vi "Main.vi"(11 "Module Admin":refnum<class "Delacor_lib_QMH_Module Admin.lvclass">) -> ()   [LabVIEW 2025, in "Data Logger v2.lvlib"]
doc: "This template is based from the Queued Message Handler design pattern and the Queued Message Handler Project Template that ships with LabVIEW 2014.\n\nThe main difference is that the Queue is private to this module and communication between modules is done via Broadcast and Request events.\n\nRequest events are wrapped via public API methods and are handled in the Event handler loop in this VI.\nAny module can register for Broadcast events sent by this module.\n\nThe Event Handling Loop generates messages based on user interface actions.\n\nThe Message Handling Loop processes messages generated by the Event Handling Loop, or by other messages. The messages are string values, so new messages can be added easily to the Message Cases case structure in the Message Handling Loop. Each message cluster can also provide an optional value for Message Data, which is a variant that can be converted to whatever message-specific data is required.\n_____\nBased on Delacor QMH Project Template 3.1.0.34.\n\n<b>Note:</b> This VI was modified by the <b>Validate DQMH Module</b> tool to call the Release Message Queue VI in the top-level Error case.\n\n<b>Note:</b> This VI was modified by the <b>Validate DQMH Module</b> tool to add a call to the Error Reported VI at the end of the 'Exit' MHL frame.\n\n<b>Note:</b> This VI was modified by the <b>Validate DQMH Module</b> tool to wrap the FP.Open method in the module close code with a Conditional Disable Structure so it does not execute when the Main VI is running as a built EXE."
uses:
  Data Logger v2.lvlib
  <vilib>/Delacor/Delacor QMH/Libraries/Module Admin_class/Delacor_lib_QMH_Module Admin.lvclass
  <vilib>/MGI/Panel Manager/Panel/Panel/Panel.lvclass
  <vilib>/Utility/miscctls.llb/LVPointTypeDef.ctl
  Module Data--cluster.ctl
  <vilib>/Delacor/Delacor QMH/Libraries/Message Queue_class/Delacor_lib_QMH_Message Queue.lvclass/Delacor_lib_QMH_Message Queue.ctl
  Stop Argument--cluster.ctl
  <vilib>/Delacor/Delacor QMH/Libraries/Module Admin_class/Delacor_lib_QMH_Module Admin.lvclass/Delacor_lib_QMH_Module Admin.ctl
  Create New TDMS Log File Argument--cluster.ctl
  Write 2D Array to TDMS Log File Argument--cluster.ctl
  Write TDMS 2D Array Parameters--cluster.ctl
  Close TDMS File Argument--cluster.ctl
  Write TDMS 2D String Array Argument--cluster.ctl
  Write TDMS 2D String Array Parameters--cluster.ctl
  Set Root Folder Path Argument--cluster.ctl
  Create New TDMS Log File (Relative Path) Argument--cluster.ctl
  Set Properties Argument--cluster.ctl
  <vilib>/Delacor/Delacor QMH/Libraries/Message Queue_class/Delacor_lib_QMH_Enqueue Message (Single).vi
  <vilib>/Delacor/Delacor QMH/Libraries/Module Admin_class/Delacor_lib_QMH_Get External Launch.vi
  <vilib>/Utility/error.llb/Error Cluster From Error Code.vi
  <vilib>/ErrorRing/Error Ring.xnode
  <vilib>/Delacor/Delacor QMH/Libraries/Message Queue_class/Delacor_lib_QMH_Message Queue.lvclass
  <vilib>/MGI/Panel Manager/Panel/Panel Helper/Panel Helper.lvclass
panel:
  in  "Panel":refnum<class "Panel.lvclass">
  in  "Simulate MHL Error":bool
  in  "Simulate EHL Error":bool
  out "error out":errorcluster
  out "Status":string
  # "Other QMH Modules communicate with this Module via its Public API (wrappers for its Request Events).\n\nThis Module communicates with other Modules via its Broadcast Events.\nAny module that wants to get these messages, just registers for this module's Broadcast events."
  # "This is a template that creates a DQMH Singleton using the MGI Panel Manager Framwork.\n\nImplement your user interface on this front panel. The Panel Manager Framework will manage showing and hiding the panel in the appropriate spot. \n\nSee the block diagram for more information on how to use this template."
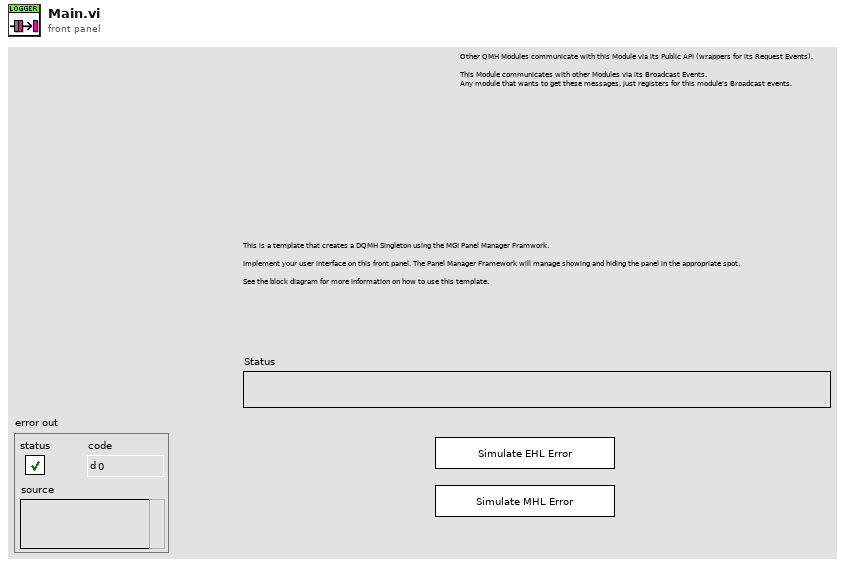
[diagram p1: front panel]
types:
  T1 = typedef "LVPointTypeDef.ctl" = cluster{"Horizontal":i16, "Vertical":i16}
  T2 = typedef "Data Logger v2.lvlib/Request Events--cluster.ctl" = cluster{"Stop Module":refnum<user-event>, "Show Panel":refnum<user-event>, "Hide Panel":refnum<user-event>, "Get Module Execution Status":refnum<user-event>, "Show Diagram":refnum<user-event>, "Change Panel":refnum<user-event>, "Create New TDMS Log File":refnum<user-event>, "Write 2D Array to TDMS Log File":refnum<user-event>, "Close TDMS File":refnum<user-event>, "Write TDMS 2D String Array":refnum<user-event>, "Set Root Folder Path":refnum<user-event>, "Create New TDMS Log File (Relative Path)":refnum<user-event>, "Set Properties":refnum<user-event>}
  T3 = typedef "Panel.lvlib/Panel Helper.lvclass/Panel Events.ctl" = cluster{"My Panel":refnum<user-event>, "Top Level Initialized":refnum<user-event>}
  T4 = typedef "Data Logger v2.lvlib/Module Data--cluster.ctl" = cluster{"Status":string, "tdms file":refnum<k34>, "State":enum16{"Idle", "Logging"}, "Root Folder Path":path}
  T5 = typedef "Data Logger v2.lvlib/Stop Argument--cluster.ctl" = cluster{"Origin":string, "Exit via Stop Module Req?":bool, "Wait for Module to stop?":bool}
  T6 = typedef "Data Logger v2.lvlib/Create New TDMS Log File Argument--cluster.ctl" = cluster{"File Path (inc. Filename)":path}
  T7 = typedef "Data Logger v2.lvlib/Write 2D Array to TDMS Log File Argument--cluster.ctl" = cluster{"TDMS Write 2D Array Parameters":T8}
  T8 = typedef "Data Logger v2.lvlib/Write TDMS 2D Array Parameters--cluster.ctl" = cluster{"Group":string, "Channel Names":string[], "Data":dbl[][]}
  T9 = typedef "Data Logger v2.lvlib/Close TDMS File Argument--cluster.ctl" = cluster{"Boolean":bool}
  T10 = typedef "Data Logger v2.lvlib/Write TDMS 2D String Array Argument--cluster.ctl" = cluster{"TDMS Write 2D String Array Parameters":T11}
  T11 = typedef "Data Logger v2.lvlib/Write TDMS 2D String Array Parameters--cluster.ctl" = cluster{"Group":string, "Channel Names":string[], "Data":string[][]}
  T12 = typedef "Data Logger v2.lvlib/Set Root Folder Path Argument--cluster.ctl" = cluster{"Root Folder Path":path}
  T13 = typedef "Data Logger v2.lvlib/Create New TDMS Log File (Relative Path) Argument--cluster.ctl" = cluster{"Filename":string}
  T14 = typedef "Data Logger v2.lvlib/Set Properties Argument--cluster.ctl" = cluster{"Property names":string[], "Property values":variant[], "Group name":string, "Channel name":string}
  T15 = enum32{"invalid lock state", "Not Locked", "Locked (No Password)", "Password-protected"}
  T16 = enum16{"open", "open or create", "create or replace", "create", "open (read-only)"}
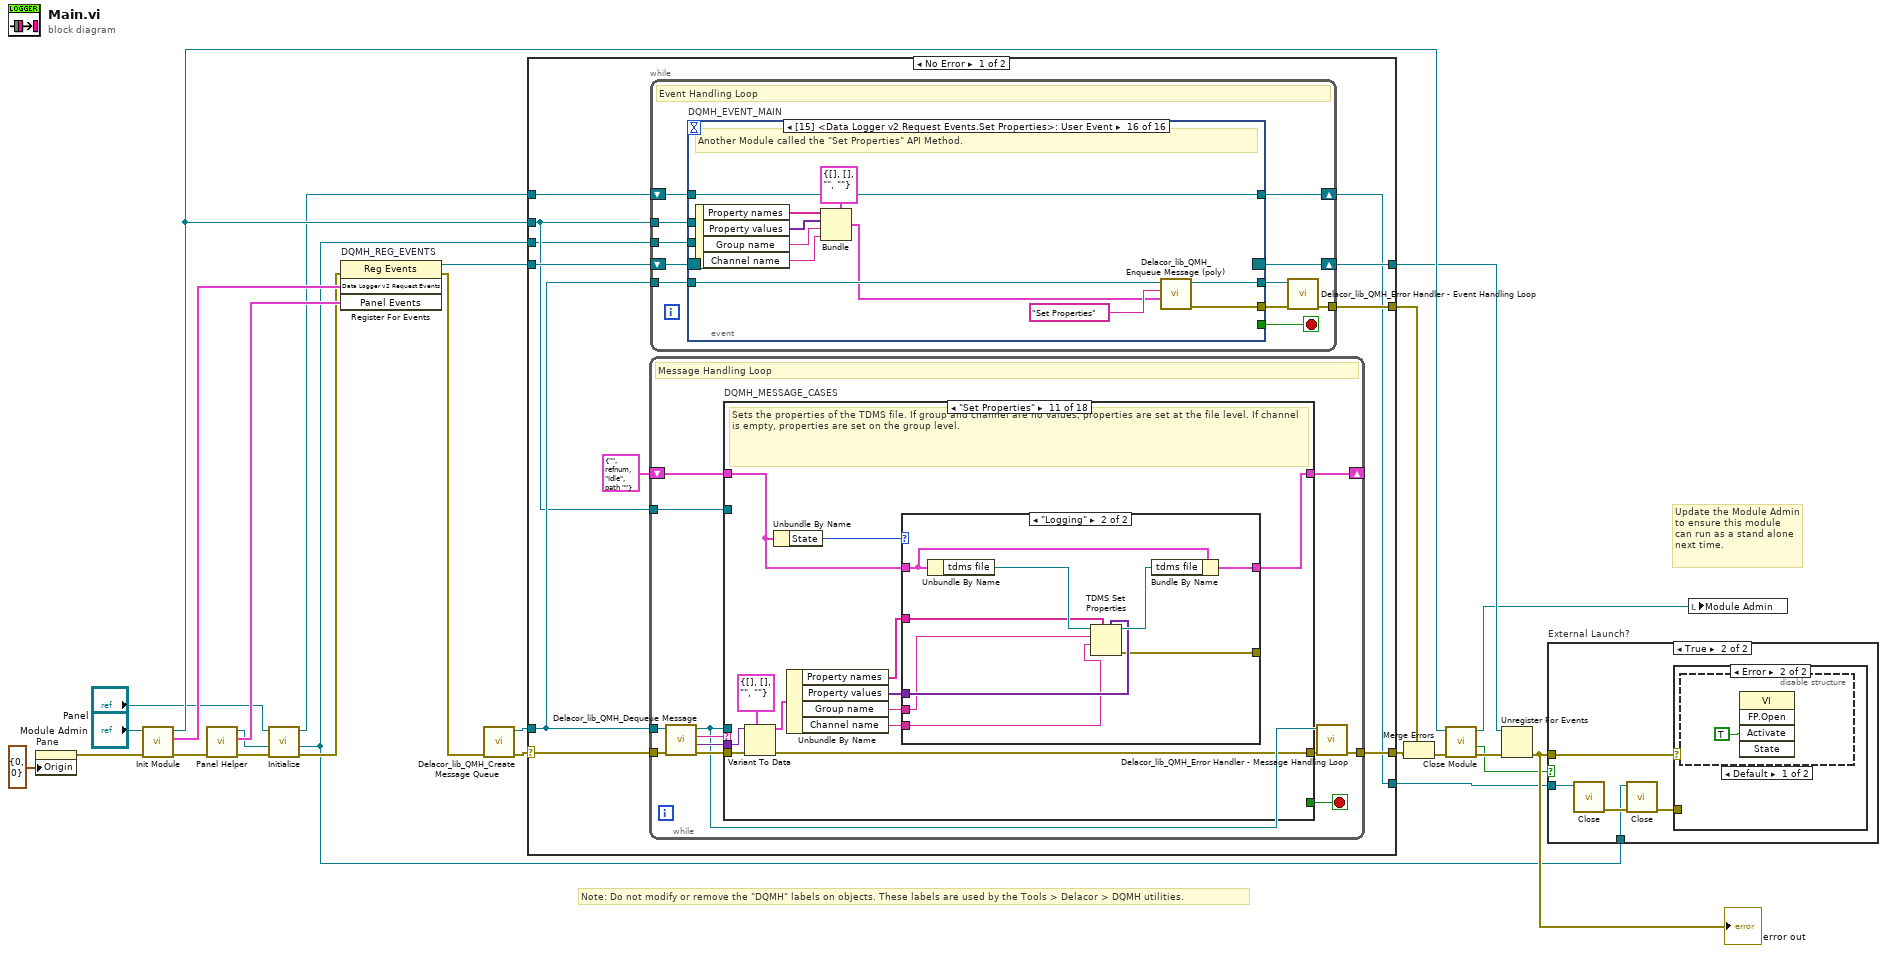
[diagram p0: block diagram]
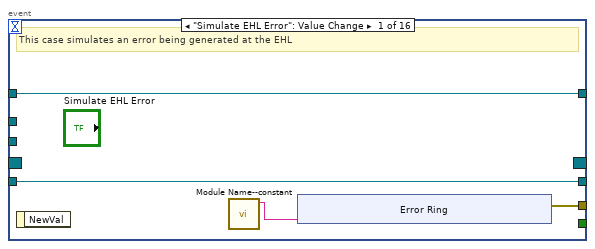
[diagram p5: hidden frame]
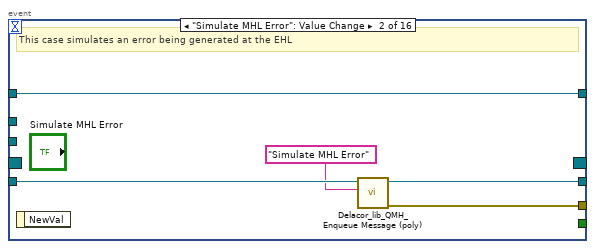
[diagram p6: hidden frame]
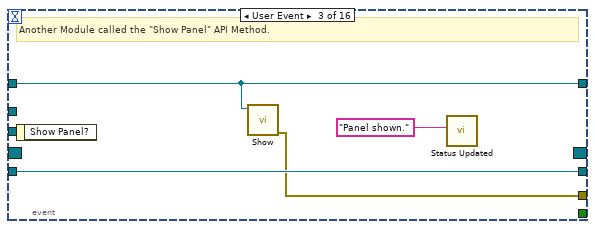
[diagram p7: hidden frame]
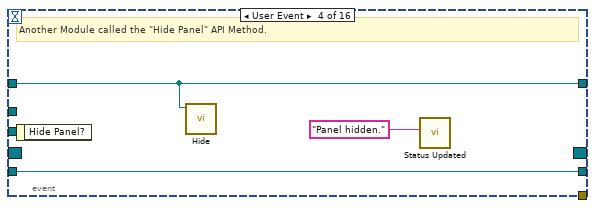
[diagram p8: hidden frame]
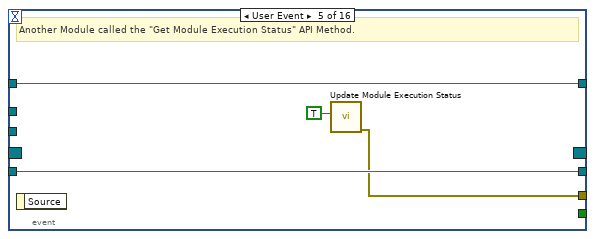
[diagram p9: hidden frame]
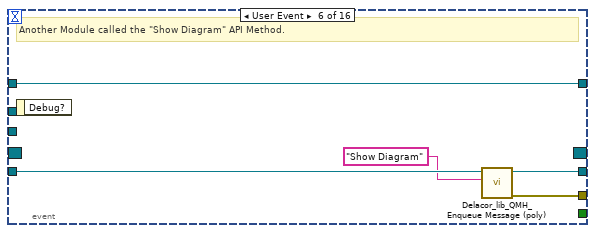
[diagram p10: hidden frame]
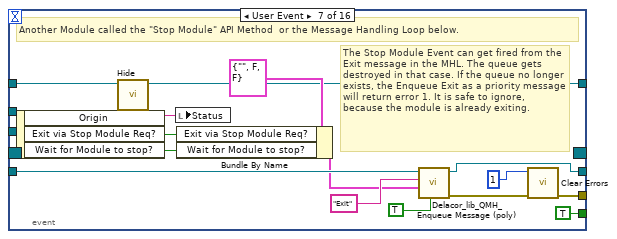
[diagram p11: hidden frame]
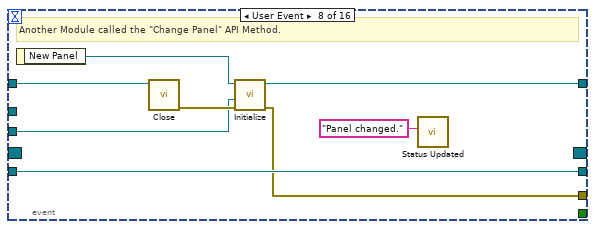
[diagram p12: hidden frame]
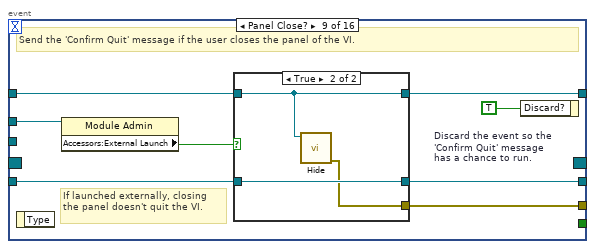
[diagram p13: hidden frame]
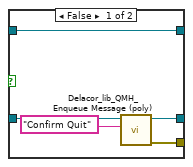
[diagram p14: hidden frame]
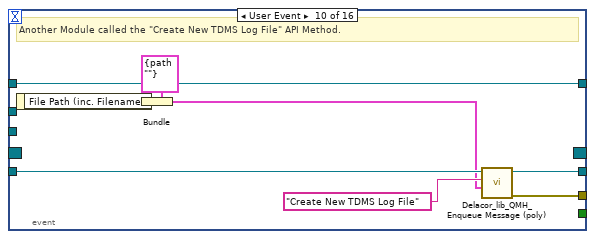
[diagram p15: hidden frame]
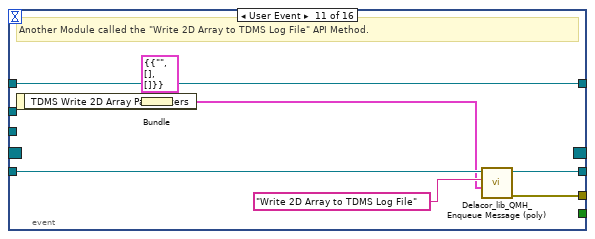
[diagram p16: hidden frame]
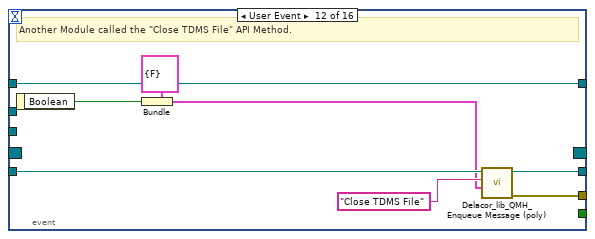
[diagram p17: hidden frame]
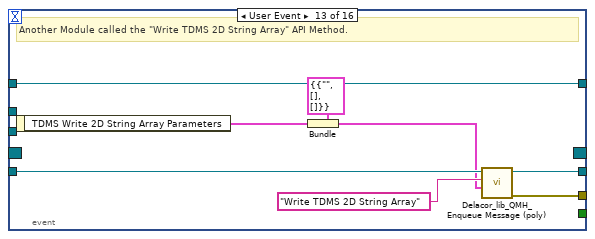
[diagram p18: hidden frame]
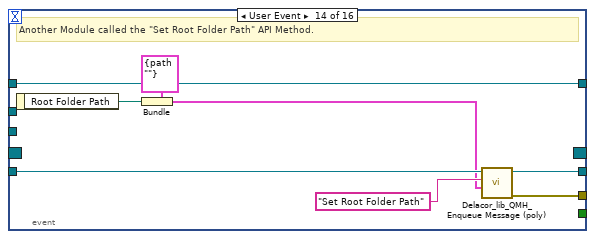
[diagram p19: hidden frame]
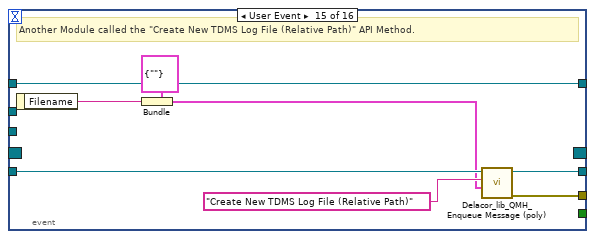
[diagram p20: hidden frame]
diagram:
  # "Note: Do not modify or remove the \"DQMH\" labels on objects. These labels are used by the Tools > Delacor > DQMH utilities."
  # "Update the Module Admin to ensure this module can run as a stand alone next time."
  n1 = property on="Pane" class="Pane"("Origin"=T1 {"Horizontal"=0, "Vertical"=0}) -> (error out=w1:errorcluster)  [unwired: 2 in, 1 out]
  n2 = call "Init Module.vi"("error in (no error)"=w1, "Singleton Module Admin in"="Module Admin") -> ("error out"=w11:errorcluster, "Data Logger v2 Request Events"=w22:T2, "Singleton Module Admin out"=w26:refnum<class "Delacor_lib_QMH_Module Admin.lvclass">)  [unwired: 7 in]
  n3 = call <vilib>:"Panel Helper.vi"("Error In"=w11) -> ("Error Out"=w8:errorcluster, "Panel Events"=w10:T3, "Panel Helper out"=w7:refnum<class "Panel Helper.lvclass">)  [unwired: 8 in]
  n4 = call <vilib>:"Initialize.vi"("error in (no error)"=w8, "My Helper in"=w7, "Panel In"="Panel") -> ("error out"=w5:errorcluster, "My Helper out"=w4:refnum<class "Panel Helper.lvclass">, "Panel Out"=w3:refnum<class "Panel.lvclass">)  [unwired: 6 in]
  n5 = register-events "DQMH_REG_EVENTS"(error in=w5, w22, w10) -> (reference out=w23:refnum<event-registration>, error out=w9:errorcluster)  [unwired: 1 in]
  n6 = call <vilib>:"Delacor_lib_QMH_Create Message Queue.vi"("error in"=w9) -> ("error out"=w13:errorcluster, "Message Queue"=w21:refnum<class "Delacor_lib_QMH_Message Queue.lvclass">)  [unwired: 9 in]
  n7 = case shown="No Error" w13 {
    selector: w13 -> [w31 w406]
    tunnel: [w37 w406] -> w25
    tunnel: [w36 w411] -> w24
    tunnel: w23 -> [w34 w411]
    tunnel: w21 -> [w33 w402]
    tunnel: [w32 _] -> w17
    tunnel: w26 -> [w30 w407]
    tunnel: w3 -> [w28 w403]
    tunnel: w4 -> [w29 _]
    tunnel: [w27 w403] -> w12
    frame No Error {
      n8 = while {
        tunnel: w33 -> [w181]
        shift-right: [w187] -> _
        shift-left: T4 {"Status"="", "tdms file"=refnum, "State"=enum."Idle", "Root Folder Path"=path ""} ("Data Cluster") -> [w188]
        tunnel: w31 -> [w185]
        tunnel: [w179] -> w37
        tunnel: w30 -> [w178]
        stop <- w186 stop-if-true
        # "Message Handling Loop"
        n9 = call-dynamic "Delacor_lib_QMH_Dequeue Message.vi"("error in"=w185, "Message Queue in"=w181) -> ("error out"=w184:errorcluster, "Message Data"=w182:variant, "Message"=w183:string, "Message Queue out"=w180:refnum<class "Delacor_lib_QMH_Message Queue.lvclass">)  [unwired: 6 in]
        n10 = case "DQMH_MESSAGE_CASES" shown="\"Set Properties\"" w183 {
          selector: w183 -> [_ _ _ _ _ _ _ _ _ _ _ _ _ _ _ _ _ w391]
          tunnel: w180 -> [_ _ _ _ _ _ _ _ _ _ _ _ _ _ w356 w371 w387 _]
          tunnel: w184 -> [w192 w204 w208 w226 w239 w249 w268 w290 w298 w312 w324 w337 w340 w345 w362 w375 w389 _]
          tunnel: [w193 w205 w207 w224 w231 w243 w267 w284 w297 w301 w323 w335 w338 w343 w353 w373 w383 w392] -> w189
          tunnel: w188 -> [w198 w206 w209 w225 w228 w241 w262 w283 w293 w300 w318 w336 w339 w344 w361 w374 w386 w393]
          tunnel: [w197 w206 w209 w225 w234 w242 w261 w282 w292 w299 w317 w336 w339 w344 w361 w374 w386 w393] -> w187
          tunnel: [_ _ _ _ _ _ _ _ _ _ _ _ _ _ _ _ w385 _] -> w186
          tunnel: w182 -> [_ w203 _ _ w238 w248 w266 w289 w296 w311 w322 _ _ _ w360 _ w382 _]
          tunnel: w178 -> [w190 _ _ _ _ _ _ _ _ _ _ _ _ _ w355 _ w376 _]
          frame "Initialize" {
            w196 = "Initial Message" ("Initial Message")
            # "#CodeNeeded - Initialize the appearance of the front panel."
            # "#CodeNeeded - Initialize your state data here."
            # "Initialize - Any operation that needs to be done before the module can receive messages. Synchronize Caller Events.vi will inform Start Module.vi that the module has launched and is ready to receive messages. Module Did Init.vi will broadcast that the module initialized."
            n11 = call "Synchronize Caller Events.vi"("error in (no error)"=w192, "Singleton Module Admin in"=w190) -> ("error out"=w191:errorcluster)  [unwired: 8 in, 1 out]
            n12 = Bundle By Name(cluster=w198, "Status"=w196) -> (w197:T4)
            n13 = local write "Status"(w196) -> ()
            n14 = call "Module Name--constant.vi"() -> ("Module Name"=w194:string)  [unwired: 11 in]
            n15 = call "Module Did Init.vi"("error in (no error)"=w191, "Initialized?"=TRUE, "Origin"=w194) -> ("error out"=w193:errorcluster)  [unwired: 8 in]
          }
          frame "Update Display" {
            # "Broadcast updated status to any VI registered to listen to this module's broadcast events."
            # "Convert the message data to a string to display in the Status indicator."
            # "#CodeRecommended - If you wish to decouple the Message Handling Loop from your user interface, consider creating User Events (like the \"Stop\" event in this VI) to message the Event Handling Loop whenever the user interface needs updating."
            # "Update Display - Update user interface here."
            n16 = Variant To Data(error in=w204, type="" ("Empty String Constant"), Variant=w203) -> (data=w201:string, error out=w200:errorcluster)
            "Status" <- w201
            n17 = call "Status Updated.vi"("error in (no error)"=w200, "Status"=w201) -> ("error out"=w199:errorcluster)  [unwired: 9 in]
            n18 = Merge Errors(w199) -> (w205:errorcluster)
          }
          frame "Show Diagram" {
            # "Show Diagram - Show the block diagram of this VI. Used as a debugging tool. There is a button in the module tester that fires the Show Diagram request, which runs this message. Note that the diagram will not be displayed if it is password-protected and the password is not in the cache."
            n19 = disable-structure shown="RUN_TIME_ENGINE==False" {
              disable-tunnel: [w217 w223] -> w207
              disable-tunnel: w208 -> [w216 w223]
              frame condition #0 (active) {
                # "functionality not available in exe"
                n20 = invoke class="VI" method="Lock State.Get"(error in=w216) -> (error out=w215:errorcluster, "Get Lock State"=w214:T15, "pwd in cache"=w211:bool)  [unwired: 3 in, 1 out]
                n21 = Equal?(x=T15."Password-protected", y=w214) -> (x = y?=w212:bool)
                n22 = Compound Arithmetic op=AND(w212, invert w211) -> (w210:bool)
                n23 = case shown="False" w210 {
                  tunnel: [w220 w222] -> w217
                  tunnel: w215 -> [w218 w222]
                  frame False {
                    n24 = property class="VI"(error in=w218, "BDWin.Open"=TRUE ("Block Diagram Window:Open")) -> (error out=w220:errorcluster)  [unwired: 1 in, 1 out]
                    n25 = call "Status Updated.vi"("Status"="Block Diagram shown." ("format string")) -> ()  [unwired: 10 in, 1 out]
                  }
                  frame True {
                    # "Password-protected VI, and the password is not in the cache. Do not show the diagram."
                  }
                }
              }
              frame condition #1 {
              }
            }
          }
          frame "--- Module Specific ---" {
            # "Separator -- The following cases handle messages specific to this Module."
            n26 = Merge Errors(w226) -> (w224:errorcluster)
          }
          frame "Create New TDMS Log File" {
            # "Creates a new TDMS log file."
            n27 = Variant To Data(error in=w239, type=T6 {"File Path (inc. Filename)"=path ""} ("Create New TDMS Log File Argument"), Variant=w238) -> (data=w236:T6, error out=w232:errorcluster)
            n28 = Unbundle By Name(w236) -> ("File Path (inc. Filename)"=w227:path)
            n29 = TDMS Open(10:T16."create or replace" ("operation (0:open)"), 11:w227) -> (0:w230:errorcluster, 3:w233:refnum<k34>)  [unwired: 5 in]
            n30 = Bundle By Name(cluster=w228, "State"=enum16{"Idle", "Logging"}."Logging", "tdms file"=w233) -> (w234:T4)
            n31 = Merge Errors(w230, w232) -> (w231:errorcluster)
          }
          frame "Write 2D Array to TDMS Log File" {
            # "Writes a 2D array to the TDMS log file."
            n32 = Variant To Data(error in=w249, type=T7 {"TDMS Write 2D Array Parameters"={"Group"="", "Channel Names"=[], "Data"=[]}} ("Write 2D Array to TDMS Log File Argument"), Variant=w248) -> (data=w246:T7, error out=w244:errorcluster)
            n33 = Unbundle By Name(w241) -> ("State"=w240:enum16{"Idle", "Logging"})
            n34 = case shown="\"Logging\"" w240 {
              tunnel: w246 -> [_ w260]
              tunnel: [errorcluster {"status"=FALSE, "code"=0, "source"=""} ("error out") w255] -> w245
              tunnel: w241 -> [w251 w254]
              tunnel: [w251 w252] -> w242
              frame "Idle", Default {
              }
              frame "Logging" {
                n35 = Unbundle By Name(w260) -> ("TDMS Write 2D Array Parameters.Group"=w258:string, "TDMS Write 2D Array Parameters.Channel Names"=w257:string[], "TDMS Write 2D Array Parameters.Data"=w256:dbl[][])
                n36 = Unbundle By Name(w254) -> ("tdms file"=w259:refnum<k34>)
                n37 = TDMS Write(0:w259, 5:w258, 7:w257, 9:w256) -> (4:w253:refnum<k34>, 15:w255:errorcluster)  [unwired: 2 in, 2 out]
                n38 = Bundle By Name(cluster=w254, "tdms file"=w253) -> (w252:T4)
              }
            }
            n39 = Merge Errors(w245, w244) -> (w243:errorcluster)
          }
          frame "Write TDMS 2D String Array" {
            # "Writes a 2D String Array to the TDMS file."
            n40 = Variant To Data(error in=w268, type=T10 {"TDMS Write 2D String Array Parameters"={"Group"="", "Channel Names"=[], "Data"=[]}} ("Write TDMS 2D String Array Argument"), Variant=w266) -> (data=w263:T10, error out=w267:errorcluster)
            n41 = Unbundle By Name(w262) -> ("State"=w264:enum16{"Idle", "Logging"})
            n42 = case shown="\"Logging\"" w264 {
              tunnel: w263 -> [_ w279]
              tunnel: [errorcluster {"status"=FALSE, "code"=0, "source"=""} ("error out") w274] -> _
              tunnel: w262 -> [w270 w273]
              tunnel: [w270 w271] -> w261
              frame "Idle", Default {
              }
              frame "Logging" {
                n43 = Unbundle By Name(w279) -> ("TDMS Write 2D String Array Parameters.Group"=w277:string, "TDMS Write 2D String Array Parameters.Channel Names"=w276:string[], "TDMS Write 2D String Array Parameters.Data"=w275:string[][])
                n44 = Unbundle By Name(w273) -> ("tdms file"=w278:refnum<k34>)
                n45 = TDMS Write(0:w278, 5:w277, 7:w276, 9:w275) -> (4:w272:refnum<k34>, 15:w274:errorcluster)  [unwired: 2 in, 2 out]
                n46 = Bundle By Name(cluster=w273, "tdms file"=w272) -> (w271:T4)
              }
            }
          }
          frame "Close TDMS File" {
            # "Closes the TDMS file."
            n47 = Variant To Data(error in=w290, type=T9 {"Boolean"=FALSE} ("Close TDMS File Argument"), Variant=w289) -> (error out=w286:errorcluster)  [unwired: 1 out]
            n48 = Unbundle By Name(w283) -> ("tdms file"=w287:refnum<k34>)
            n49 = TDMS Close(8:w286, 11:w287) -> (0:w285:errorcluster)  [unwired: 1 out]
            n50 = call <vilib>:"Clear Errors.vi"("error in (no error)"=w285) -> ("error out"=w284:errorcluster)  [unwired: 5 in, 1 out]
            n51 = Bundle By Name(cluster=w283, "State"=enum16{"Idle", "Logging"}."Idle", "tdms file"=refnum<k34> refnum) -> (w282:T4)
          }
          frame "Set Root Folder Path" {
            # "Sets the root folder path."
            n52 = Variant To Data(error in=w298, type=T12 {"Root Folder Path"=path ""} ("Set Root Folder Path Argument"), Variant=w296) -> (data=w294:T12, error out=w297:errorcluster)
            n53 = Unbundle By Name(w294) -> ("Root Folder Path"=w291:path)
            n54 = Bundle By Name(cluster=w293, "Root Folder Path"=w291) -> (w292:T4)
          }
          frame "Create New TDMS Log File (Relative Path)" {
            # "Creates a New TDMS with a relative path."
            n55 = Variant To Data(error in=w312, type=T13 {"Filename"=""} ("Create New TDMS Log File (Relative Path) Argument"), Variant=w311) -> (data=w309:T13, error out=w302:errorcluster)
            n56 = Unbundle By Name(w300) -> ("Root Folder Path"=w305:path)
            n57 = Unbundle By Name(w309) -> ("Filename"=w304:string)
            n58 = Build Path(base path=w305, name or relative path=w304) -> (appended path=w303:path)
            n59 = TDMS Open(8:w302, 10:T16."create or replace" ("operation (0:open)"), 11:w303) -> (0:w301:errorcluster, 3:w307:refnum<k34>)  [unwired: 4 in]
            n60 = Bundle By Name(cluster=w300, "State"=enum16{"Idle", "Logging"}."Logging", "tdms file"=w307) -> (w299:T4)
          }
          frame "Set Properties" {
            # "Sets the properties of the TDMS file. If group and channel are no values, properties are set at the file level. If channel is empty, properties are set on the group level."
            n61 = Variant To Data(error in=w324, type=T14 {"Property names"=[], "Property values"=[], "Group name"="", "Channel name"=""} ("Set Properties Argument"), Variant=w322) -> (data=w320:T14, error out=w323:errorcluster)
            n62 = Unbundle By Name(w318) -> ("State"=w319:enum16{"Idle", "Logging"})
            n63 = Unbundle By Name(w320) -> ("Property names"=w316:string[], "Property values"=w315:variant[], "Group name"=w314:string, "Channel name"=w313:string)
            n64 = case shown="\"Logging\"" w319 {
              tunnel: w318 -> [w325 w326]
              tunnel: [w325 w332] -> w317
              tunnel: w316 -> [_ w331]
              tunnel: w315 -> [_ w330]
              tunnel: w314 -> [_ w329]
              tunnel: w313 -> [_ w328]
              tunnel: [_ w327] -> _
              frame "Idle", Default {
              }
              frame "Logging" {
                n65 = Unbundle By Name(w326) -> ("tdms file"=w334:refnum<k34>)
                n66 = TDMS Set Properties(5:w330, 7:w331, 9:w328, 10:w329, 11:w334) -> (0:w327:errorcluster, 3:w333:refnum<k34>)  [unwired: 1 in, 2 out]
                n67 = Bundle By Name(cluster=w326, "tdms file"=w333) -> (w332:T4)
              }
            }
          }
          frame "---Copy This Frame---" {
            # "Duplicate this frame when creating new messages.  Change this comment in the duplicated frame to describe this message."
            n68 = Merge Errors(w337) -> (w335:errorcluster)
          }
          frame "--- Exit and Error Handling---" {
            # "Separator - The following cases handle errors and exit messages."
            n69 = Merge Errors(w340) -> (w338:errorcluster)
          }
          frame "Simulate MHL Error" {
            # "Simulate an error occurring at the MHL"
            n70 = call "Module Name--constant.vi"() -> ("Module Name"=w342:string)  [unwired: 11 in]
            n71 = xnode "Error Ring"("parameter 0"=w342) -> ("error out"=w341:errorcluster)
            n72 = Merge Errors(w345, w341) -> (w343:errorcluster)
          }
          frame "Error" {
            # "#CodeRecommended - If you ever change the name of this \"Error\" message, you'll need to update the name in the Check Loop Error.vi as well."
            # "#CodeRecommended - If the module is running in standalone mode (External Launch = FALSE), this code will pop up an error dialog and call the 'Exit' message if an error occurs. Add more fine-grained error handling here."
            # "Error - Check the error message data and respond accordingly. This message is sent by the \"Error Handler\" VIs at the end of each loop in this application."
            n73 = property class="Module Admin"(reference=w355) -> ("Accessors:External Launch"=w354:bool)  [unwired: 1 in, 2 out]
            n74 = Variant To Data(error in=w362, type=errorcluster {"status"=FALSE, "code"=0, "source"=""} ("error constant"), Variant=w360) -> (data=w363:errorcluster, error out=w358:errorcluster)
            n75 = call "Error Reported.vi"("Error"=w363) -> ()  [unwired: 10 in, 1 out]
            n76 = case shown="False" w354 {
              tunnel: [w368 _] -> w357
              tunnel: w356 -> [w367 _]
              tunnel: w363 -> [w364 _]
              frame False {
                # "If the module is running standalone, then pop up an error dialog and call the \"Exit\" message."
                n77 = call <vilib>:"Simple Error Handler.vi"("error in (no error)"=w364) -> ()  [unwired: 4 in, 5 out]
                n78 = call-poly <vilib>:"Delacor_lib_QMH_Enqueue Message (poly).vi"("Priority Message? (F)"=TRUE, "Message"="Exit", "Message Queue in"=w367) -> ("error out"=w368:errorcluster)  [unwired: 7 in, 1 out]
              }
              frame True {
                # "If the module was launched externally, calling the Error Reported broadcast VI is the only action performed by the \"Error\" message. The module's caller can then process the error appropriately."
              }
            }
            n79 = Merge Errors(w358, w357) -> (w353:errorcluster)
            n80 = local write "error out"(w353) -> ()
          }
          frame "Confirm Quit" {
            # "#CodeNeeded - If you want to provide an \"Are you sure\" dialog (or some other notification) before the application exits, place that code here. This message is typically sent from a Panel Close? event."
            # "Confirm Quit - Message that can confirm whether or not the user wants to exit the application."
            n81 = call-poly <vilib>:"Delacor_lib_QMH_Enqueue Message (poly).vi"("Priority Message? (F)"=TRUE, "error in"=w375, "Message"="Exit", "Message Queue in"=w371) -> ("error out"=w372:errorcluster)  [unwired: 6 in, 1 out]
            n82 = Merge Errors(w372) -> (w373:errorcluster)
          }
          frame "Exit" {
            w380 = 91  # 91: not all Exit messages will have an argument
            w385 = TRUE  # Stop the VI
            # "Release the message queue reference"
            # "#CodeNeeded - Add any required cleanup code here"
            # "Exit - Exit the application."
            n83 = Variant To Data(error in=w389, type=T5 {"Origin"="", "Exit via Stop Module Req?"=FALSE, "Wait for Module to stop?"=FALSE} ("Stop Argument"), Variant=w382) -> (data=w378:T5, error out=w381:errorcluster)
            n84 = call <vilib>:"Clear Errors.vi"("error in (no error)"=w381, "specific error code to clear (0: all)"=w380) -> ("error out"=w388:errorcluster)  [unwired: 4 in, 1 out]
            n85 = call-dynamic "Delacor_lib_QMH_Release Message Queue.vi"("error in"=w388, "Message Queue"=w387) -> ("error out"=w384:errorcluster)  [unwired: 9 in]
            n86 = call "Handle Exit.vi"("Stop Argument"=w378, "Admin in"=w376) -> ("error out"=w377:errorcluster)  [unwired: 8 in, 1 out]
            n87 = Merge Errors(w377, w384) -> (w383:errorcluster)
            n88 = call "Error Reported.vi"("Error"=w383) -> ()  [unwired: 10 in, 1 out]
          }
          frame Default {
            # "'Default' case only runs if there is a message that isn't defined in any of the other cases.  Output a programming error."
            n89 = call "Module Name--constant.vi"() -> ("Module Name"=w390:string)  [unwired: 11 in]
            n90 = xnode "Error Ring"("parameter 0"=w391, "parameter 1"=w390) -> ("error out"=w392:errorcluster)
          }
        }
        n91 = call-dynamic "Delacor_lib_QMH_Error Handler - Message Handling Loop.vi"("error in"=w189, "Message Queue in"=w180) -> ("dup error in"=w179:errorcluster)  [unwired: 8 in, 1 out]
      }
      n92 = while {
        tunnel: w33 -> [w48]
        shift-right: [w46] -> w36
        shift-left: w34 -> [w47]
        tunnel: [w42] -> w32
        tunnel: w30 -> [w41]
        tunnel: w29 -> [w40]
        shift-right: [w38] -> w27
        shift-left: w28 -> [w39]
        stop <- w44 stop-if-true
        # "Event Handling Loop"
        n93 = event "DQMH_EVENT_MAIN" shown="[15] <Data Logger v2 Request Events.Set Properties>: User Event" {
          selector: w47 -> [_ _ _ _ _ _ _ _ _ _ _ _ _ _ _ _]
          dyn-events: [_ _ _ _ _ _ _ _ _ _ _ _ _ _ _ _] -> w46
          timeout: _ -> [_ _ _ _ _ _ _ _ _ _ _ _ _ _ _ _]
          tunnel: [_ _ _ _ _ _ TRUE ("Discard?") _ _ _ _ _ _ _ _ _] -> w44
          tunnel: w48 -> [w52 w64 w68 w71 w75 w80 w92 w102 w109 w126 w134 w142 w150 w158 w166 w177]
          tunnel: [w51 w61 w66 _ w74 w77 w86 w98 w108 w119 w127 w135 w143 w151 w159 w167] -> w45
          tunnel: [w52 w63 w68 w71 w75 w79 w91 w102 w107 w124 w132 w140 w148 w156 w164 w175] -> w43
          tunnel: w41 -> [_ _ _ _ _ _ _ _ w106 _ _ _ _ _ _ _]
          tunnel: w40 -> [_ _ _ _ _ _ _ w97 _ _ _ _ _ _ _ _]
          tunnel: w39 -> [w49 w60 w67 w70 w72 w76 w81 w101 w104 w125 w133 w141 w149 w157 w165 w176]
          tunnel: [w49 w60 w67 w70 w72 w76 w81 w96 w103 w125 w133 w141 w149 w157 w165 w176] -> w38
          event "Simulate EHL Error": Value Change {
            # "This case simulates an error being generated at the EHL"
            n94 = event-data() -> ()  [unwired: 1 in, 1 out]
            n95 = call "Module Name--constant.vi"() -> ("Module Name"=w50:string)  [unwired: 11 in]
            n96 = xnode "Error Ring"("parameter 0"=w50) -> ("error out"=w51:errorcluster)
          }
          event "Simulate MHL Error": Value Change {
            # "This case simulates an error being generated at the EHL"
            n97 = event-data() -> ()  [unwired: 1 in, 1 out]
            n98 = call-poly <vilib>:"Delacor_lib_QMH_Enqueue Message (poly).vi"("Message"="Simulate MHL Error", "Message Queue in"=w64) -> ("error out"=w61:errorcluster, "Message Queue out"=w63:refnum<class "Delacor_lib_QMH_Message Queue.lvclass">)  [unwired: 8 in]
          }
          event User Event {
            # "Another Module called the \"Show Panel\" API Method."
            n99 = event-data() -> ()  [unwired: 1 in, 1 out]
            n100 = call <vilib>:"Show.vi"("Panel in"=w67) -> ("Error Out"=w66:errorcluster)  [unwired: 10 in]
            n101 = call "Status Updated.vi"("Status"="Panel shown." ("format string")) -> ()  [unwired: 10 in, 1 out]
          }
          event User Event {
            # "Another Module called the \"Hide Panel\" API Method."
            n102 = event-data() -> ()  [unwired: 1 in, 1 out]
            n103 = call <vilib>:"Hide.vi"("Panel In"=w70) -> ()  [unwired: 10 in, 1 out]
            n104 = call "Status Updated.vi"("Status"="Panel hidden." ("format string")) -> ()  [unwired: 10 in, 1 out]
          }
          event User Event {
            # "Another Module called the \"Get Module Execution Status\" API Method."
            n105 = event-data() -> ()  [unwired: 1 in, 1 out]
            n106 = call "Update Module Execution Status.vi"("Running?"=TRUE) -> ("error out"=w74:errorcluster)  [unwired: 10 in]
          }
          event User Event {
            # "Another Module called the \"Show Diagram\" API Method."
            n107 = event-data() -> ()  [unwired: 1 in, 1 out]
            n108 = call-poly <vilib>:"Delacor_lib_QMH_Enqueue Message (poly).vi"("Message"="Show Diagram", "Message Queue in"=w80) -> ("error out"=w77:errorcluster, "Message Queue out"=w79:refnum<class "Delacor_lib_QMH_Message Queue.lvclass">)  [unwired: 8 in]
          }
          event User Event {
            # "The Stop Module Event can get fired from the Exit message in the MHL. The queue gets destroyed in that case. If the queue no longer exists, the Enqueue Exit as a priority message will return error 1. It is safe to ignore, because the module is already exiting."
            # "Another Module called the \"Stop Module\" API Method  or the Message Handling Loop below."
            n109 = event-data() -> ("Origin"=w90:string, "Exit via Stop Module Req?"=w84:bool, "Wait for Module to stop?"=w83:bool)  [unwired: 1 in]
            n110 = call <vilib>:"Hide.vi"("Panel In"=w81) -> ()  [unwired: 10 in, 1 out]
            n111 = local write "Status"(w90) -> ()
            n112 = Bundle By Name(cluster=T5 {"Origin"="", "Exit via Stop Module Req?"=FALSE, "Wait for Module to stop?"=FALSE} ("Stop Argument"), "Exit via Stop Module Req?"=w84, "Wait for Module to stop?"=w83) -> (w82:T5)
            n113 = call-poly <vilib>:"Delacor_lib_QMH_Enqueue Message (poly).vi"("Priority Message? (F)"=TRUE, "Message Data"=w82, "Message"="Exit", "Message Queue in"=w92) -> ("error out"=w87:errorcluster, "Message Queue out"=w91:refnum<class "Delacor_lib_QMH_Message Queue.lvclass">)  [unwired: 6 in]
            n114 = call <vilib>:"Clear Errors.vi"("error in (no error)"=w87, "specific error code to clear (0: all)"=1) -> ("error out"=w86:errorcluster)  [unwired: 4 in, 1 out]
          }
          event User Event {
            # "Another Module called the \"Change Panel\" API Method."
            n115 = event-data() -> ("New Panel"=w100:refnum<class "Panel.lvclass">)  [unwired: 1 in]
            n116 = call-dynamic <vilib>:"Close.vi"("Panel In"=w101) -> ("Error Out"=w99:errorcluster)  [unwired: 10 in]
            n117 = call <vilib>:"Initialize.vi"("error in (no error)"=w99, "My Helper in"=w97, "Panel In"=w100) -> ("error out"=w98:errorcluster, "Panel Out"=w96:refnum<class "Panel.lvclass">)  [unwired: 6 in, 1 out]
            n118 = call "Status Updated.vi"("Status"="Panel changed.") -> ()  [unwired: 10 in, 1 out]
          }
          event Panel Close? {
            w110 = TRUE  # Discard the event so the 'Confirm Quit' message has a chance to run.
            # "If launched externally, closing the panel doesn't quit the VI."
            # "Send the 'Confirm Quit' message if the user closes the panel of the VI."
            n119 = event-data() -> ()  [unwired: 1 in, 1 out]
            n120 = property class="Module Admin"(reference=w106) -> ("Accessors:External Launch"=w105:bool)  [unwired: 1 in, 2 out]
            n121 = case shown="True" w105 {
              tunnel: w109 -> [w115 w118]
              tunnel: [w114 w116] -> w108
              tunnel: [w113 w118] -> w107
              tunnel: w104 -> [w111 w117]
              tunnel: [w111 w117] -> w103
              frame False {
                n122 = call-poly <vilib>:"Delacor_lib_QMH_Enqueue Message (poly).vi"("Message"="Confirm Quit", "Message Queue in"=w115) -> ("error out"=w114:errorcluster, "Message Queue out"=w113:refnum<class "Delacor_lib_QMH_Message Queue.lvclass">)  [unwired: 8 in]
              }
              frame True {
                n123 = call <vilib>:"Hide.vi"("Panel In"=w117) -> ("Error Out"=w116:errorcluster)  [unwired: 10 in]
              }
            }
            n124 = event-data("Discard?"=w110) -> ()  [unwired: 1 in, 1 out]
          }
          event User Event {
            # "Another Module called the \"Create New TDMS Log File\" API Method."
            n125 = event-data() -> ("File Path (inc. Filename)"=w120:path)  [unwired: 1 in]
            n126 = Bundle(cluster=T6 {"File Path (inc. Filename)"=path ""} ("Create New TDMS Log File Argument"), "File Path (inc. Filename)"=w120) -> (w121:T6)
            n127 = call-poly <vilib>:"Delacor_lib_QMH_Enqueue Message (poly).vi"("Message Data"=w121, "Message"="Create New TDMS Log File", "Message Queue in"=w126) -> ("error out"=w119:errorcluster, "Message Queue out"=w124:refnum<class "Delacor_lib_QMH_Message Queue.lvclass">)  [unwired: 7 in]
          }
          event User Event {
            # "Another Module called the \"Write 2D Array to TDMS Log File\" API Method."
            n128 = event-data() -> ("TDMS Write 2D Array Parameters"=w128:T8)  [unwired: 1 in]
            n129 = Bundle(cluster=T7 {"TDMS Write 2D Array Parameters"={"Group"="", "Channel Names"=[], "Data"=[]}} ("Write 2D Array to TDMS Log File Argument"), "TDMS Write 2D Array Parameters"=w128) -> (w129:T7)
            n130 = call-poly <vilib>:"Delacor_lib_QMH_Enqueue Message (poly).vi"("Message Data"=w129, "Message"="Write 2D Array to TDMS Log File", "Message Queue in"=w134) -> ("error out"=w127:errorcluster, "Message Queue out"=w132:refnum<class "Delacor_lib_QMH_Message Queue.lvclass">)  [unwired: 7 in]
          }
          event User Event {
            # "Another Module called the \"Close TDMS File\" API Method."
            n131 = event-data() -> ("Boolean"=w136:bool)  [unwired: 1 in]
            n132 = Bundle(cluster=T9 {"Boolean"=FALSE} ("Close TDMS File Argument"), "Boolean"=w136) -> (w137:T9)
            n133 = call-poly <vilib>:"Delacor_lib_QMH_Enqueue Message (poly).vi"("Message Data"=w137, "Message"="Close TDMS File", "Message Queue in"=w142) -> ("error out"=w135:errorcluster, "Message Queue out"=w140:refnum<class "Delacor_lib_QMH_Message Queue.lvclass">)  [unwired: 7 in]
          }
          event User Event {
            # "Another Module called the \"Write TDMS 2D String Array\" API Method."
            n134 = event-data() -> ("TDMS Write 2D String Array Parameters"=w144:T11)  [unwired: 1 in]
            n135 = Bundle(cluster=T10 {"TDMS Write 2D String Array Parameters"={"Group"="", "Channel Names"=[], "Data"=[]}} ("Write TDMS 2D String Array Argument"), "TDMS Write 2D String Array Parameters"=w144) -> (w145:T10)
            n136 = call-poly <vilib>:"Delacor_lib_QMH_Enqueue Message (poly).vi"("Message Data"=w145, "Message"="Write TDMS 2D String Array", "Message Queue in"=w150) -> ("error out"=w143:errorcluster, "Message Queue out"=w148:refnum<class "Delacor_lib_QMH_Message Queue.lvclass">)  [unwired: 7 in]
          }
          event User Event {
            # "Another Module called the \"Set Root Folder Path\" API Method."
            n137 = event-data() -> ("Root Folder Path"=w152:path)  [unwired: 1 in]
            n138 = Bundle(cluster=T12 {"Root Folder Path"=path ""} ("Set Root Folder Path Argument"), "Root Folder Path"=w152) -> (w153:T12)
            n139 = call-poly <vilib>:"Delacor_lib_QMH_Enqueue Message (poly).vi"("Message Data"=w153, "Message"="Set Root Folder Path", "Message Queue in"=w158) -> ("error out"=w151:errorcluster, "Message Queue out"=w156:refnum<class "Delacor_lib_QMH_Message Queue.lvclass">)  [unwired: 7 in]
          }
          event User Event {
            # "Another Module called the \"Create New TDMS Log File (Relative Path)\" API Method."
            n140 = event-data() -> ("Filename"=w160:string)  [unwired: 1 in]
            n141 = Bundle(cluster=T13 {"Filename"=""} ("Create New TDMS Log File (Relative Path) Argument"), "Filename"=w160) -> (w161:T13)
            n142 = call-poly <vilib>:"Delacor_lib_QMH_Enqueue Message (poly).vi"("Message Data"=w161, "Message"="Create New TDMS Log File (Relative Path)", "Message Queue in"=w166) -> ("error out"=w159:errorcluster, "Message Queue out"=w164:refnum<class "Delacor_lib_QMH_Message Queue.lvclass">)  [unwired: 7 in]
          }
          event User Event {
            # "Another Module called the \"Set Properties\" API Method."
            n143 = event-data() -> ("Property names"=w171:string[], "Property values"=w170:variant[], "Group name"=w169:string, "Channel name"=w168:string)  [unwired: 1 in]
            n144 = Bundle(cluster=T14 {"Property names"=[], "Property values"=[], "Group name"="", "Channel name"=""} ("Set Properties Argument"), "Property names"=w171, "Property values"=w170, "Group name"=w169, "Channel name"=w168) -> (w172:T14)
            n145 = call-poly <vilib>:"Delacor_lib_QMH_Enqueue Message (poly).vi"("Message Data"=w172, "Message"="Set Properties", "Message Queue in"=w177) -> ("error out"=w167:errorcluster, "Message Queue out"=w175:refnum<class "Delacor_lib_QMH_Message Queue.lvclass">)  [unwired: 7 in]
          }
        }
        n146 = call-dynamic "Delacor_lib_QMH_Error Handler - Event Handling Loop.vi"("error in"=w45, "Message Queue in"=w43) -> ("dup error in"=w42:errorcluster)  [unwired: 8 in, 1 out]
      }
    }
    frame Error {
      # "Synchronize Caller Events.vi will inform Start Module.vi that the module has launched and will let the code calling Start Module.vi register for broadcasts and would permit the caller receive the broadcast that an error occurred at launch time."
      n147 = call-dynamic "Delacor_lib_QMH_Release Message Queue.vi"("Message Queue"=w402) -> ()  [unwired: 10 in, 1 out]
      n148 = call "Synchronize Caller Events.vi"("Singleton Module Admin in"=w407) -> ("error out"=w404:errorcluster)  [unwired: 9 in, 1 out]
      n149 = call "Module Name--constant.vi"() -> ("Module Name"=w410:string)  [unwired: 11 in]
      n150 = Format Into String(format string="An error occurred during initialization. %s is no longer running.", w410) -> (resulting string=w408:string)  [unwired: 2 in, 1 out]
      n151 = Merge Errors(w406, w404) -> (w405:errorcluster)
      n152 = call "Error Reported.vi"("Additional Information"=w408, "Error"=w405) -> ()  [unwired: 9 in, 1 out]
    }
  }
  n153 = Merge Errors(w17, w25) -> (w16:errorcluster)
  n154 = call "Close Module.vi"("error in (no error)"=w16, "Module Admin in"=w26) -> ("error out"=w19:errorcluster, "External Launch"=w14:bool, "Module Admin out"=w18:refnum<class "Delacor_lib_QMH_Module Admin.lvclass">)  [unwired: 7 in]
  n155 = Unregister For Events(event registration refnum=w24, error in=w19) -> (error out=w15:errorcluster)
  "error out" <- w15
  n156 = case "External Launch?" shown="True" w14 {
    tunnel: w15 -> [_ w416]
    tunnel: w12 -> [_ w415]
    tunnel: w4 -> [_ w413]
    frame False {
    }
    frame True {
      n157 = call-dynamic <vilib>:"Close.vi"("Panel In"=w415) -> ("Error Out"=w414:errorcluster)  [unwired: 10 in]
      n158 = call <vilib>:"Close.vi"("error in (no error)"=w414, "Controller in"=w413) -> ("error out"=w412:errorcluster)  [unwired: 9 in]
      n159 = case shown="Error" w416 {
        tunnel: w412 -> [_ _]
        frame No Error {
        }
        frame Error {
          n160 = disable-structure shown="Default" {
            frame condition #0 (active) {
              n161 = invoke class="VI" method="FP.Open"("Activate"=TRUE ("Activate?")) -> ()  [unwired: 4 in, 5 out]
            }
            frame condition #1 {
              # "Don't show panel on error if running inside a built EXE."
            }
          }
        }
      }
    }
  }
  n162 = local write "Module Admin"(w18) -> ()
